vi "BRig_RT__calc_Tvalley.vi"(7 "input_peakWidth":dbl, 10 "input_freq":dbl) -> (2 "output_Tvalley":dbl)   [LabVIEW 2014]
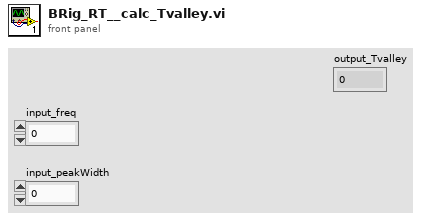
[diagram p1: front panel]
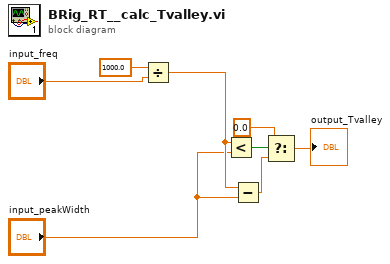
[diagram p0: block diagram]
diagram:
  n1 = Divide(x=1000.0, y="input_freq") -> (x/y=w4:dbl)
  n2 = Less?(x=w4, y="input_peakWidth") -> (x < y?=w6:bool)
  n3 = Subtract(x=w4, y="input_peakWidth") -> (x-y=w2:dbl)
  n4 = Select(t=0.0, s=w6, f=w2) -> (s? t:f=→"output_Tvalley":dbl)
